vi "manual_trigger.vi"() -> ()   [LabVIEW 2011]
panel:
  in  "cont. trigger":bool
  out "trigger number":i32
  in  "cont. trigger":bool
  in  "milliseconds to wait":u32=100
  in  "number of triggers":i32
  in  "single trigger":bool
  in  "stop":bool
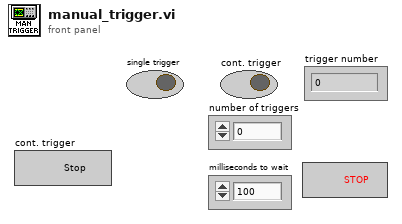
[diagram p1: front panel]
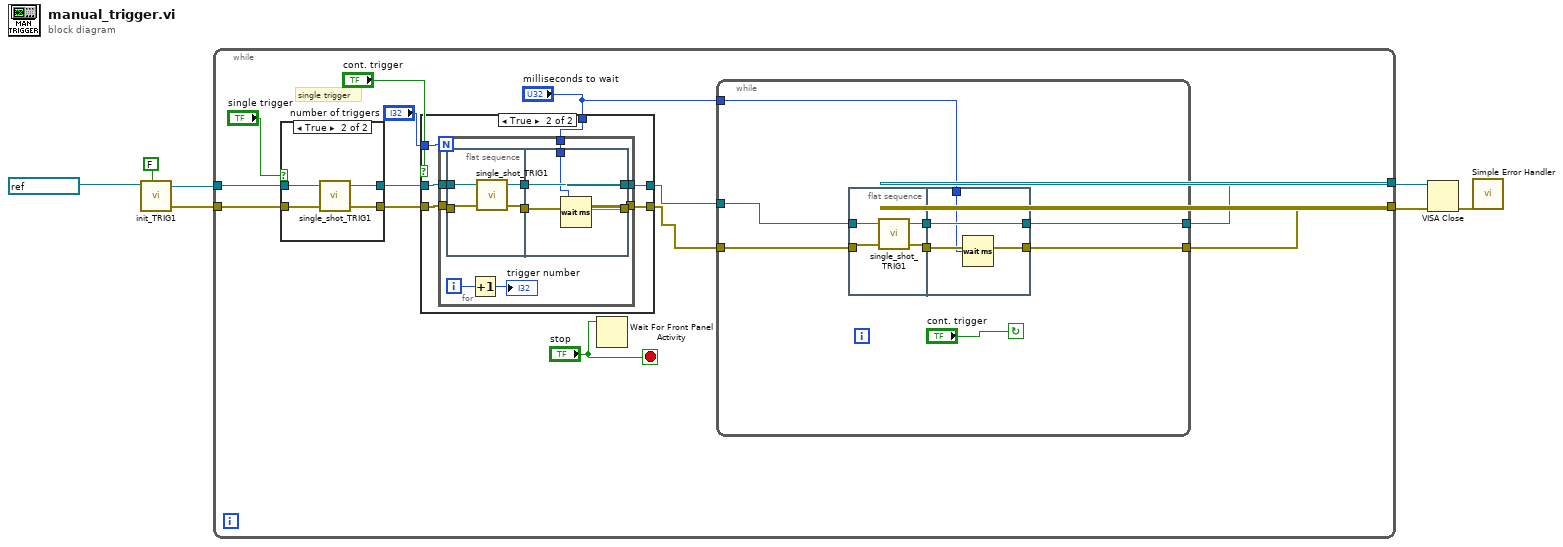
[diagram p0: block diagram]
diagram:
  n1 = call "init_TRIG1.vi"("reset"=FALSE ("reset TRIG"), "VISA resource name"=refnum<visa-resource-name> "TRIG1") -> ("error out"=w6:errorcluster, "VISA resource name out"=w7:refnum<visa-resource-name>)  [unwired: 8 in]
  n2 = while {
    tunnel: w7 -> [w18]
    tunnel: w6 -> [w17]
    tunnel: [w10] -> w4
    tunnel: [w9] -> w3
    stop <- "stop" stop-if-true
    # "single trigger"
    n3 = case shown="True" "single trigger" {
      tunnel: w18 -> [w37 w41]
      tunnel: w17 -> [w36 w40]
      tunnel: [w37 w39] -> w16
      tunnel: [w36 w38] -> w15
      frame False {
      }
      frame True {
        n4 = call "single_shot_TRIG1.vi"("error in (no error)"=w40, "VISA resource name"=w41) -> ("error out"=w38:errorcluster, "VISA resource name 2"=w39:refnum<visa-resource-name>)  [unwired: 2 in]
      }
    }
    n5 = case shown="True" "cont. trigger" {
      tunnel: w16 -> [w43 w49]
      tunnel: w15 -> [w42 w48]
      tunnel: [w43 w47] -> w12
      tunnel: [w42 w46] -> w11
      tunnel: "number of triggers" -> [_ w45]
      tunnel: "milliseconds to wait" -> [_ w44]
      frame False {
      }
      frame True {
        n6 = for {
          N: w45 -> [_]
          tunnel: w49 -> [w58]
          tunnel: w48 -> [w57]
          tunnel: [w56] -> w47
          tunnel: [w55] -> w46
          tunnel: w44 -> [w52]
          i -> [w51]
          n7 = flat-sequence {
            tunnel: w58 -> [w62]
            tunnel: w57 -> [w61]
            tunnel: [w60] -> w54
            tunnel: [w59] -> w53
            tunnel: [w64] -> w55
            tunnel: [w65] -> w56
            tunnel: w54 -> [w65]
            tunnel: w53 -> [w64]
            tunnel: w52 -> [w63]
            frame #0 {
              n8 = call "single_shot_TRIG1.vi"("error in (no error)"=w61, "VISA resource name"=w62) -> ("error out"=w59:errorcluster, "VISA resource name 2"=w60:refnum<visa-resource-name>)  [unwired: 2 in]
            }
            frame #1 {
              n9 = Wait (ms)(milliseconds to wait=w63) -> ()  [unwired: 1 out]
            }
          }
          n10 = Increment(x=w51) -> (x+1=→"trigger number":i32)
        }
      }
    }
    n11 = Wait For Front Panel Activity(3:"stop") -> ()  [unwired: 2 in, 1 out]
    n12 = while {
      tunnel: w12 -> [w25]
      tunnel: w11 -> [w24]
      tunnel: [w23] -> w10
      tunnel: [w22] -> w9
      tunnel: "milliseconds to wait" -> [w21]
      stop <- "cont. trigger" continue-if-true
      n13 = flat-sequence {
        tunnel: w25 -> [w32]
        tunnel: w24 -> [w31]
        tunnel: [w30] -> w28
        tunnel: [w29] -> w27
        tunnel: [w34] -> w22
        tunnel: [w35] -> w23
        tunnel: w28 -> [w35]
        tunnel: w27 -> [w34]
        tunnel: w21 -> [w33]
        frame #0 {
          n14 = call "single_shot_TRIG1.vi"("error in (no error)"=w31, "VISA resource name"=w32) -> ("error out"=w29:errorcluster, "VISA resource name 2"=w30:refnum<visa-resource-name>)  [unwired: 2 in]
        }
        frame #1 {
          n15 = Wait (ms)(milliseconds to wait=w33) -> ()  [unwired: 1 out]
        }
      }
    }
  }
  n16 = VISA Close(VISA resource name=w4, error in (no error)=w3) -> (error out=w5:errorcluster)
  n17 = call <vilib>:"Simple Error Handler.vi"("error in (no error)"=w5) -> ()  [unwired: 4 in, 5 out]
